vi "StartMessageReceiver.vi"(8 "error in (no error)":errorcluster, 11 "STOMP in":refnum<class "STOMP.lvclass">) -> (0 "error out":errorcluster, 3 "STOMP out":refnum<class "STOMP.lvclass">)   [LabVIEW 2017, in "LabVIEW STOMP.lvlib" / "STOMP.lvclass"]
uses:
  STOMP.lvclass
  MessageReceiver.vi
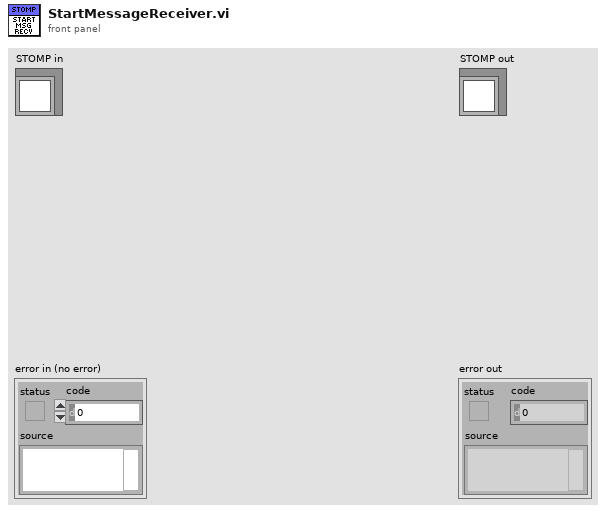
[diagram p1: front panel]
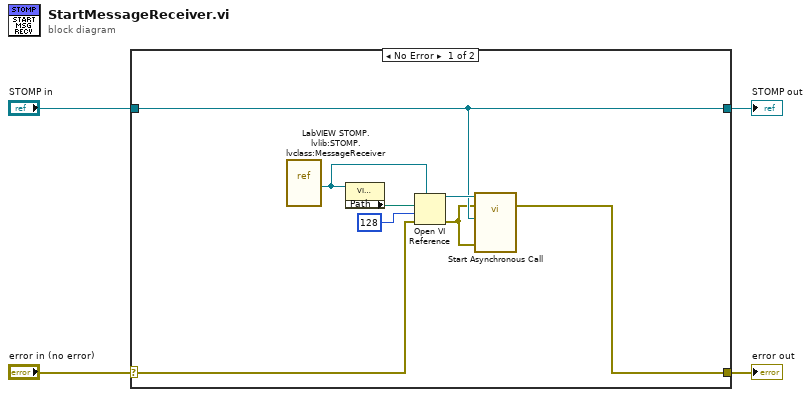
[diagram p0: block diagram]
diagram:
  n1 = case shown="No Error" "error in (no error)" {
    selector: "error in (no error)" -> [w6 w14]
    tunnel: [w5 w14] -> w3
    tunnel: [w8 w13] -> w1
    tunnel: "STOMP in" -> [w8 w13]
    frame No Error {
      n2 = vi-ref "LabVIEW STOMP.lvlib:STOMP.lvclass:MessageReceiver.vi"() -> (w11:refnum<vi>)
      n3 = property class="VI (strict)"(reference=w11) -> ("Path"=w12:path)  [unwired: 1 in, 2 out]
      n4 = Open VI Reference(type specifier VI Refnum (for type only)=w11, vi path=w12, options=128, error in (no error)=w6) -> (vi reference=w9:refnum<vi>, error out=w7:errorcluster)  [unwired: 2 in]
      n5 = call-by-ref "Start Asynchronous Call"(reference=w9, error in=w7, "STOMP In"=w8, 5:"error in (no error)"=w7) -> (error out=w5:errorcluster)  [unwired: 17 in, 2 out]
    }
    frame Error {
    }
  }
  "error out" <- w3
  "STOMP out" <- w1
